vi "Read Custom Device VI.vi"(8 "Error In":errorcluster caption="error in", 11 "Custom Device .NET Ref In":refnum<k24>) -> (0 "Error Out":errorcluster caption="error in", 2 "Supported Targets Properties":T1, 3 "Custom Device .NET Ref In":refnum<k24>)   [LabVIEW 2019, in "VeriStand Custom Device XML Parser.lvlib"]
doc: "Reads and returns the properties of all supported targets"
uses:
  VeriStand Custom Device XML Parser.lvlib
  NationalInstruments.VeriStand.XMLReader
  XML Controls/Custom Device Source Distribution Properties.ctl
  XML Controls/Path Cluster.ctl
  XML Controls/Supported Targets.ctl
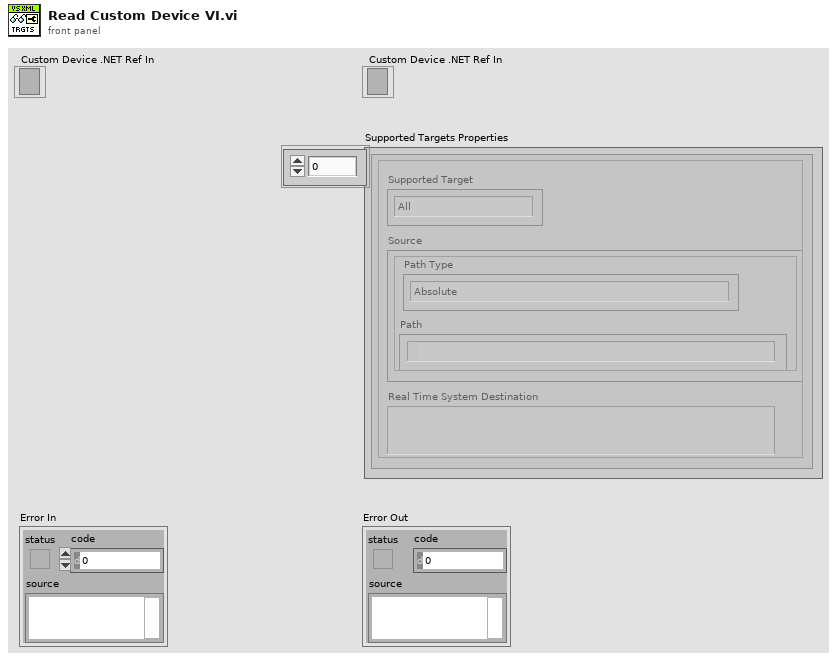
[diagram p1: front panel]
types:
  T1 = typedef "VeriStand Custom Device XML Parser.lvlib/Custom Device Source Distribution Properties.ctl" = cluster{"Source":T2, "Real Time System Destination":string, "Supported Target":T3}[]
  T2 = typedef "VeriStand Custom Device XML Parser.lvlib/Path Cluster.ctl" = cluster{"Path":path, "Path Type":enum16{"Absolute", "To Base", "To Common Doc Dir", "To Application Data Dir"}}
  T3 = typedef "VeriStand Custom Device XML Parser.lvlib/Supported Targets.ctl" = enum16{"All", "Pharlap", "VxWorks", "Windows", "Linux_32_ARM", "Linux_x64", "PharlapWindows", "PharlapVxWorks", "VxWorksWindows"}
  T4 = cluster{"Source":T2, "Real Time System Destination":string, "Supported Target":T3}
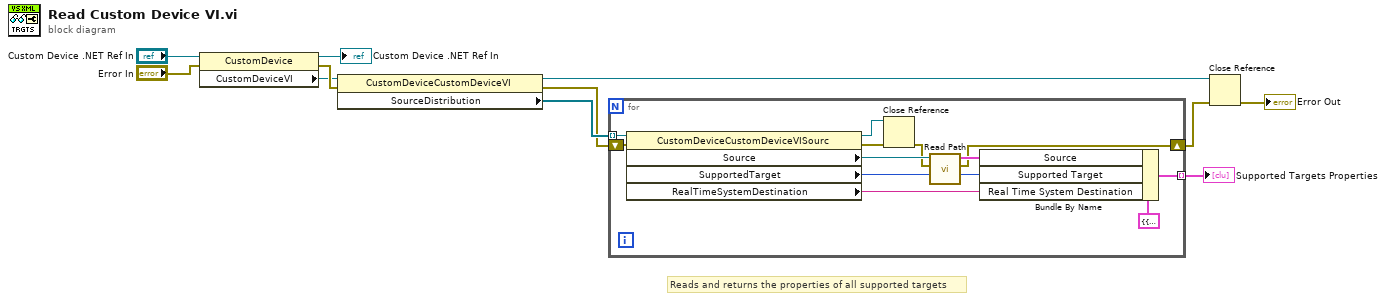
[diagram p0: block diagram]
diagram:
  # "Reads and returns the properties of all supported targets"
  n1 = property class="CustomDevice"(reference="Custom Device .NET Ref In", error in="Error In") -> (reference out=→"Custom Device .NET Ref In":refnum<k24>, error out=w9:errorcluster, "CustomDeviceVI"=w8:refnum<k24>)
  n2 = property class="CustomDeviceCustomDeviceVI"(reference=w8, error in=w9) -> (reference out=w4:refnum<k24>, error out=w5:errorcluster, "SourceDistribution"=w7:refnum<k24>[])
  n3 = for {
    tunnel: w7 -> [w23] mode=indexing
    shift-right: [w12] -> w3
    shift-left: w5 -> [w22]
    tunnel: [w18] -> w1 mode=indexing
    n4 = property class="CustomDeviceCustomDeviceVISourc"(reference=w23, error in=w22) -> (reference out=w21:refnum<k24>, error out=w14:errorcluster, "Source"=w20:refnum<k24>, "SupportedTarget"=w17:i32, "RealTimeSystemDestination"=w19:string)
    n5 = Close Reference(reference=w21, error in (no error)=w14) -> (error out=w13:errorcluster)
    n6 = call "Read Path.vi"("Error In"=w13, "Path .NET Ref"=w20) -> ("Error Out"=w12:errorcluster, "Path Properties"=w16:T2)  [unwired: 8 in]
    n7 = Bundle By Name(cluster=T4 {"Source"={"Path"=path "", "Path Type"=enum."Absolute"}, "Real Time System Destination"="", "Supported Target"=enum."All"} ("Source"), "Source"=w16, "Supported Target"=w17, "Real Time System Destination"=w19) -> (w18:T4)
  }
  "Supported Targets Properties" <- w1
  n8 = Close Reference(reference=w4, error in (no error)=w3) -> (error out=→"Error Out":errorcluster)
